vi "subDFD_Preprocess Signal Input.vi"(6 "input quantizer":T1={"source"=1, "wl"=32, "iwl"=1, "overflow mode"=enum."Saturation", "rounding mode"=enum."Nearest", "signed?"=TRUE} {"source" items=["Coefficients a/k"=0, "Coefficients b/v"=7, "Input"=1, "Output"=2, "Multiplicand"=3, "Product"=4, "Sum"=5, "Delay"=6]}, 7 "input range":dbl=1.0, 11 "x":dbl[](array[numeric])) -> (2 "integer q[x]":i32[](array[numeric]), 3 "q[x]":dbl[](array[numeric]))   [LabVIEW 2017]
doc: "Preprocess the input floating-point signal according to the input quantizer to make sure the comparison between floating-point filtering reference and fixed-point filtering simulation is fair from the perspective of input accuracy."
uses:
  <vilib>/addons/Digital Filter Design/_Objects.llb/DFD Quantization Settings.ctl
  <vilib>/addons/Digital Filter Design/_Objects.llb/DFD Quantization Sources.ctl
  <vilib>/addons/Digital Filter Design/FXPLib.llb/DFD I32 to FXP (vector).vi
  <vilib>/addons/Digital Filter Design/FXPLib.llb/DFD FXP to I32 (vector).vi
  <vilib>/addons/Digital Filter Design/NI_DigFilterLicensed.lvlib
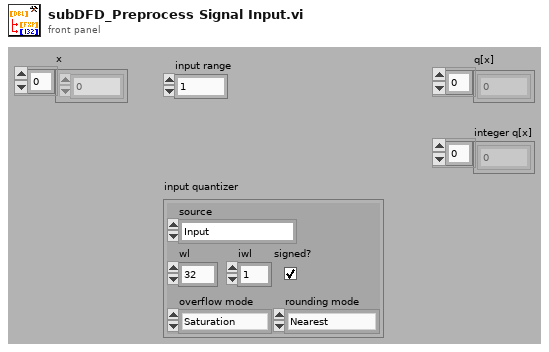
[diagram p1: front panel]
types:
  T1 = typedef "NI_DigFilterLicensed.lvlib/DFD Quantization Settings.ctl" = cluster{"source":T2, "wl":i16, "iwl":i16, "overflow mode":enum16{"Saturation", "Wrap"}, "rounding mode":enum16{"Nearest", "Truncation"}, "signed?":bool}
  T2 = typedef "NI_DigFilterLicensed.lvlib/DFD Quantization Sources.ctl" = u16
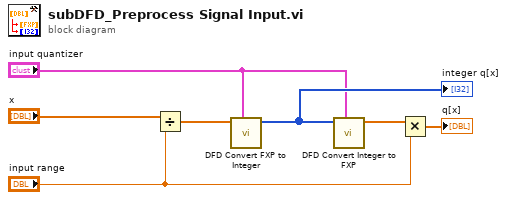
[diagram p0: block diagram]
diagram:
  n1 = Divide(x="x", y="input range") -> (x/y=w6:dbl[])
  n2 = call-poly <vilib>:"DFD Convert FXP to Integer.vi"("quantization settings"="input quantizer", "FXP values"=w6) -> ("I32 values"=w5:i32[])  [unwired: 1 in, 8 out]
  "integer q[x]" <- w5
  n3 = call-poly <vilib>:"DFD Convert Integer to FXP.vi"("quantization settings"="input quantizer", "I32 values"=w5) -> ("FXP values"=w3:dbl[])  [unwired: 1 in, 8 out]
  n4 = Multiply(x=w3, y="input range") -> (x*y=→"q[x]":dbl[])
